vi "Raise Water Level.vi"(8 "error in (no error)":errorcluster, 10 "Data":variant, 11 "App Data":T1={"Pump Station Controls"={"Lag Pump"=enum."OFF", "Lead Pump"=enum."OFF", "ALARM"=0.0, "LAG"=0.0, "LEAD"=0.0, "STOP"=0.0}, "Pump Indicators"={"Pump Water Level"=0.0, "ALARM"=FALSE, "LAG"=FALSE, "LEAD"=FALSE, "STOP"=FALSE, "PUMP 1 STATE"=FALSE, "PUMP 2 STATE"=FALSE}, "Alarm"=refnum, "Lag Start Time"=timestamp(0 s since 1904-01-01), "Lead Start Time"=timestamp(0 s since 1904-01-01), "Main Q"=refnum} {"Pump Indicators"."Pump Water Level" scale=0.0..4.0}) -> (0 "error out":errorcluster, 3 "App Data 2":T1={"Pump Station Controls"={"Lag Pump"=enum."OFF", "Lead Pump"=enum."OFF", "ALARM"=0.0, "LAG"=0.0, "LEAD"=0.0, "STOP"=0.0}, "Pump Indicators"={"Pump Water Level"=0.0, "ALARM"=FALSE, "LAG"=FALSE, "LEAD"=FALSE, "STOP"=FALSE, "PUMP 1 STATE"=FALSE, "PUMP 2 STATE"=FALSE}, "Alarm"=refnum, "Lag Start Time"=timestamp(0 s since 1904-01-01), "Lead Start Time"=timestamp(0 s since 1904-01-01), "Main Q"=refnum} {"Pump Indicators"."Pump Water Level" scale=0.0..4.0})   [LabVIEW 2024]
uses:
  App Data.ctl
  Pump Controls.ctl
  Pump Switch.ctl
  Pump Indicators.ctl
  Q Info.ctl
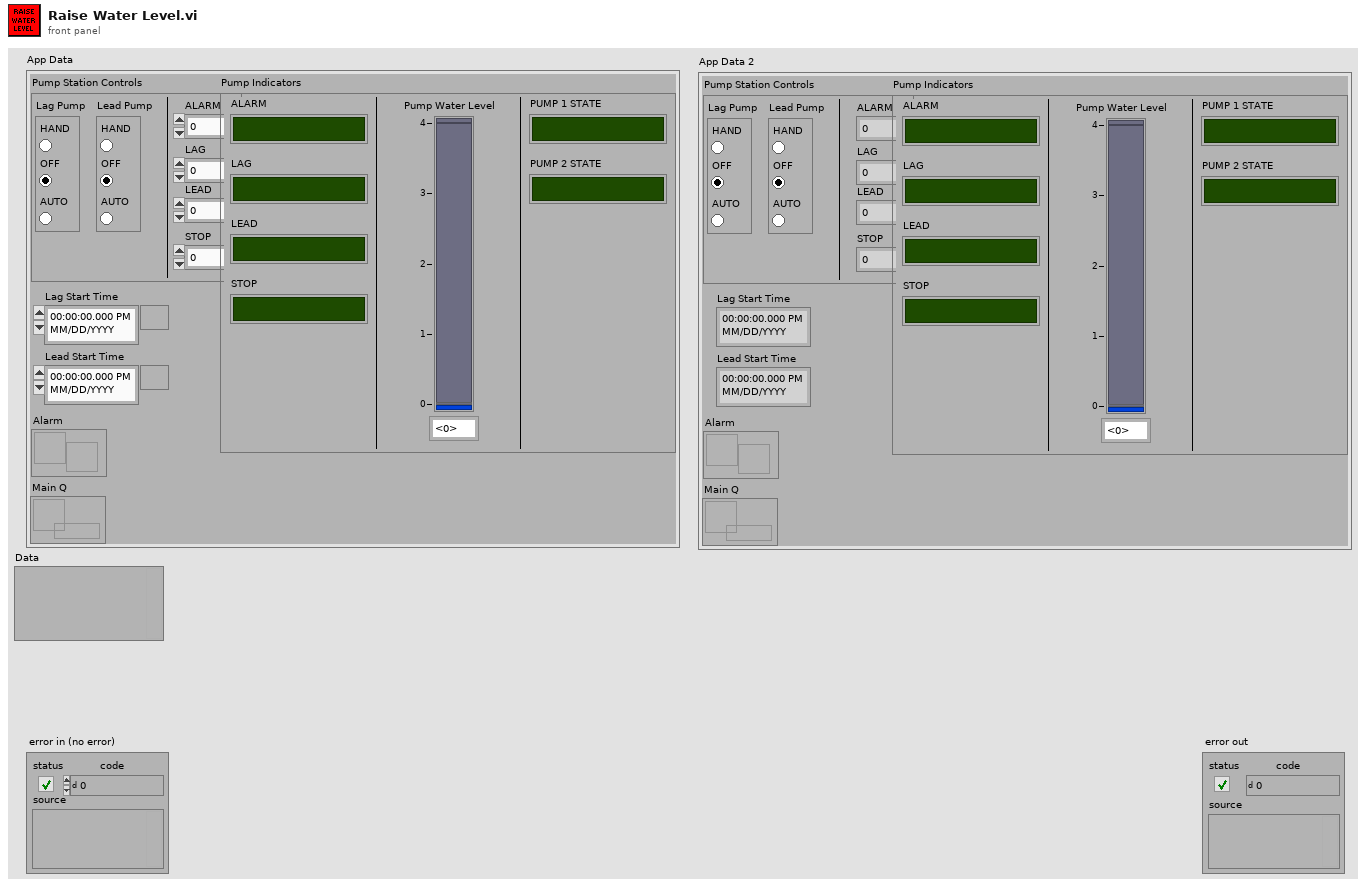
[diagram p1: front panel]
types:
  T1 = typedef "App Data.ctl" = cluster{"Pump Station Controls":T2, "Pump Indicators":T4, "Alarm":refnum<notifier>, "Lag Start Time":timestamp, "Lead Start Time":timestamp, "Main Q":refnum<queue>}
  T2 = typedef "Pump Controls.ctl" = cluster{"Lag Pump":T3, "Lead Pump":T3, "ALARM":dbl, "LAG":dbl, "LEAD":dbl, "STOP":dbl}
  T3 = typedef "Pump Switch.ctl" = enum32{"HAND", "OFF", "AUTO"}
  T4 = typedef "Pump Indicators.ctl" = cluster{"Pump Water Level":dbl, "ALARM":bool, "LAG":bool, "LEAD":bool, "STOP":bool, "PUMP 1 STATE":bool, "PUMP 2 STATE":bool}
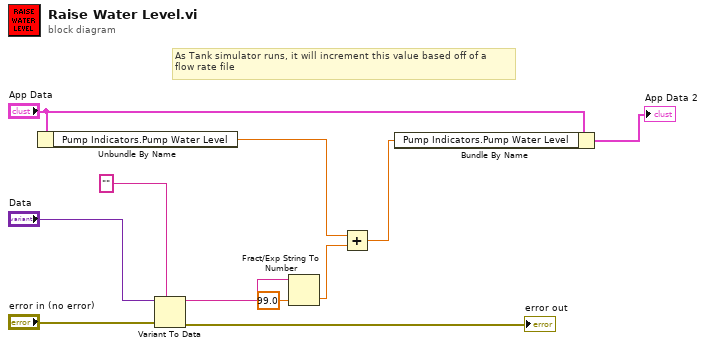
[diagram p0: block diagram]
diagram:
  # "As Tank simulator runs, it will increment this value based off of a\nflow rate file"
  n1 = Unbundle By Name("App Data") -> ("Pump Indicators.Pump Water Level"=w4:dbl)
  n2 = Variant To Data(error in="error in (no error)", type="", Variant="Data") -> (data=w8:string, error out=→"error out":errorcluster)
  n3 = Fract/Exp String To Number(string=w8, default (0 dbl)=99.0 ("default (0 DBL)")) -> (number=w5:dbl)  [unwired: 2 in, 1 out]
  n4 = Add(x=w4, y=w5) -> (x+y=w2:dbl)
  n5 = Bundle By Name(cluster="App Data", "Pump Indicators.Pump Water Level"=w2) -> (→"App Data 2":T1)
